vi "Make Connections.vi"(8 "error in (no error)":errorcluster, 10 "Enums in":refnum<vi>[](array[refnum]), 11 "Tunnel in":refnum<vi>[](array[refnum])) -> (0 "error out":errorcluster)   [LabVIEW 2019]
uses:
  VI Scripting Utilities/VI Scripting Utilities.lvlib
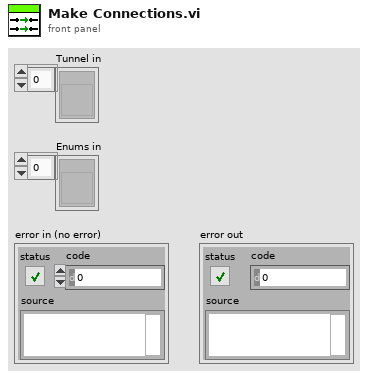
[diagram p1: front panel]
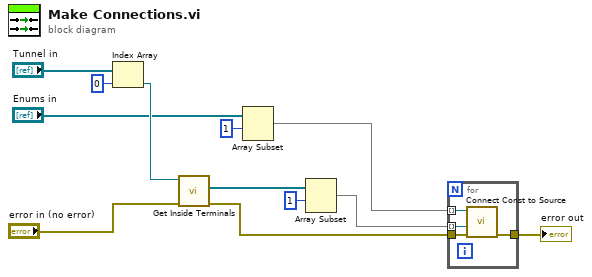
[diagram p0: block diagram]
diagram:
  n1 = Index Array(array="Tunnel in", index=0) -> (element=w9:refnum<vi>)
  n2 = call "Get Inside Terminals.vi"("Error In"="error in (no error)", "Tunnel in"=w9) -> ("Error Out"=w12:errorcluster, "InsideTerms[]"=w11:refnum<vi>[])  [unwired: 7 in, 1 out]
  n3 = Array Subset(array="Enums in", index=1) -> (w1:refnum<vi>[])  [unwired: 1 in]
  n4 = Array Subset(array=w11, index=1) -> (w5:refnum<vi>[])  [unwired: 1 in]
  n5 = for {
    tunnel: w1 -> [w15] mode=indexing
    tunnel: [w13] -> w8
    tunnel: w5 -> [w16] mode=indexing
    tunnel: w12 -> [w14]
    n6 = call "Connect Const to Source.vi"("Error In"=w14, "Source"=w16, "Const in"=w15) -> ("Error Out"=w13:errorcluster)  [unwired: 7 in, 1 out]
  }
  "error out" <- w8
